vi "TelemetryDev.vi"(8 "error in":errorcluster, 10 "ON/OFF":bool, 11 "VISA resource name in":refnum<visa-resource-name>) -> (0 "error out":errorcluster, 3 "VISA resource name out":refnum<visa-resource-name>, 4 "Laser PRR, kHz":dbl caption="Частота следования импульсов" format="%#_g kHz", 5 "Power DB-25":T1, 6 "module temp":dbl caption="Темп. модуля" format="%#_g °C", 7 "Laser Power,%":dbl caption="Мощьность, %" format="%#_g ")   [LabVIEW 2014]
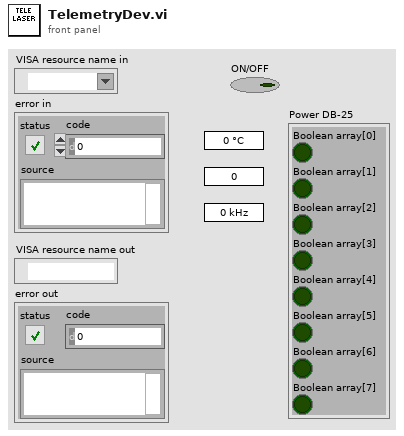
[diagram p1: front panel]
types:
  T1 = cluster{"Boolean array[0]":bool, "Boolean array[1]":bool, "Boolean array[2]":bool, "Boolean array[3]":bool, "Boolean array[4]":bool, "Boolean array[5]":bool, "Boolean array[6]":bool, "Boolean array[7]":bool}
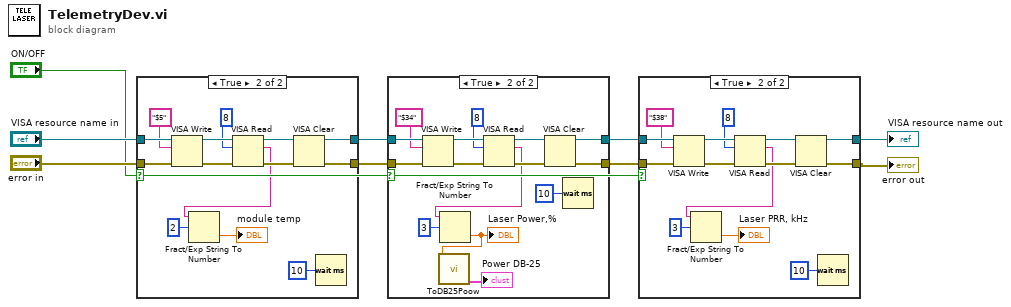
[diagram p0: block diagram]
diagram:
  n1 = case shown="True" "ON/OFF" {
    tunnel: "VISA resource name in" -> [w11 w23]
    tunnel: "error in" -> [w10 w22]
    tunnel: [w11 w18] -> w7
    tunnel: [w10 w17] -> w6
    frame False {
    }
    frame True {
      n2 = VISA Write(VISA resource name=w23, write buffer="$5", error in (no error)=w22) -> (VISA resource name out=w24:refnum<visa-resource-name>, error out=w25:errorcluster)  [unwired: 1 out]
      n3 = VISA Read(VISA resource name=w24, byte count=u32 8, error in (no error)=w25) -> (VISA resource name out=w20:refnum<visa-resource-name>, read buffer=w14:string, error out=w19:errorcluster)  [unwired: 1 out]
      n4 = Fract/Exp String To Number(string=w14, offset=2) -> (number=→"module temp":dbl)  [unwired: 2 in, 1 out]
      n5 = VISA Clear(VISA resource name=w20, error in (no error)=w19) -> (VISA resource name out=w18:refnum<visa-resource-name>, error out=w17:errorcluster)
      n6 = Wait (ms)(milliseconds to wait=u32 10) -> ()  [unwired: 1 out]
    }
  }
  n7 = case shown="True" "ON/OFF" {
    tunnel: w7 -> [w27 w40]
    tunnel: w6 -> [w26 w39]
    tunnel: [w27 w35] -> w3
    tunnel: [w26 w34] -> w2
    frame False {
    }
    frame True {
      n8 = VISA Write(VISA resource name=w40, write buffer="$34", error in (no error)=w39) -> (VISA resource name out=w41:refnum<visa-resource-name>, error out=w42:errorcluster)  [unwired: 1 out]
      n9 = VISA Read(VISA resource name=w41, byte count=u32 8, error in (no error)=w42) -> (VISA resource name out=w37:refnum<visa-resource-name>, read buffer=w31:string, error out=w36:errorcluster)  [unwired: 1 out]
      n10 = Fract/Exp String To Number(string=w31, offset=3) -> (number=w29:dbl)  [unwired: 2 in, 1 out]
      "Laser Power,%" <- w29
      n11 = call "ToDB25Poow.vi"("Power,%"=w29) -> ("cluster"=→"Power DB-25":T1)  [unwired: 10 in]
      n12 = VISA Clear(VISA resource name=w37, error in (no error)=w36) -> (VISA resource name out=w35:refnum<visa-resource-name>, error out=w34:errorcluster)
      n13 = Wait (ms)(milliseconds to wait=u32 10) -> ()  [unwired: 1 out]
    }
  }
  n14 = case shown="True" "ON/OFF" {
    tunnel: w3 -> [w44 w56]
    tunnel: w2 -> [w43 w55]
    tunnel: [w44 w51] -> w5
    tunnel: [w43 w50] -> w4
    frame False {
    }
    frame True {
      n15 = VISA Write(VISA resource name=w56, write buffer="$38", error in (no error)=w55) -> (VISA resource name out=w57:refnum<visa-resource-name>, error out=w58:errorcluster)  [unwired: 1 out]
      n16 = VISA Read(VISA resource name=w57, byte count=u32 8, error in (no error)=w58) -> (VISA resource name out=w53:refnum<visa-resource-name>, read buffer=w47:string, error out=w52:errorcluster)  [unwired: 1 out]
      n17 = Fract/Exp String To Number(string=w47, offset=3) -> (number=→"Laser PRR, kHz":dbl)  [unwired: 2 in, 1 out]
      n18 = VISA Clear(VISA resource name=w53, error in (no error)=w52) -> (VISA resource name out=w51:refnum<visa-resource-name>, error out=w50:errorcluster)
      n19 = Wait (ms)(milliseconds to wait=u32 10) -> ()  [unwired: 1 out]
    }
  }
  "VISA resource name out" <- w5
  "error out" <- w4
